vi "Write Tags.vi"(8 "error in (no error)":errorcluster, 10 "Array of Values":dbl[](array[numeric]), 11 "Communication Channel in":refnum<class "Communication Channel.lvclass">) -> (0 "error out":errorcluster, 3 "Communication Channel out":refnum<class "Communication Channel.lvclass">)   [LabVIEW 2014, in "Communication Channel.lvclass"]
uses:
  Communication Channel.lvclass
  Communication Channel.lvclass/Communication Channel.ctl
  <vilib>/Skyline/Tag/Wrapper/Wrapper_class/Write Tag (DBL).vi
  <vilib>/Skyline/Tag/Wrapper/Wrapper_class/NI Skyline Tag.lvclass
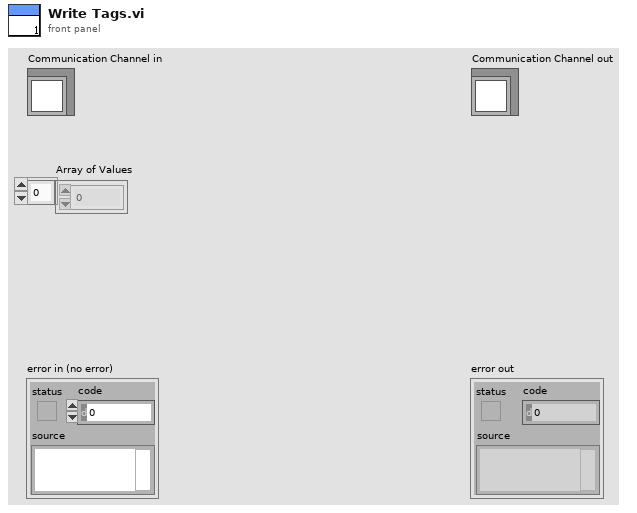
[diagram p1: front panel]
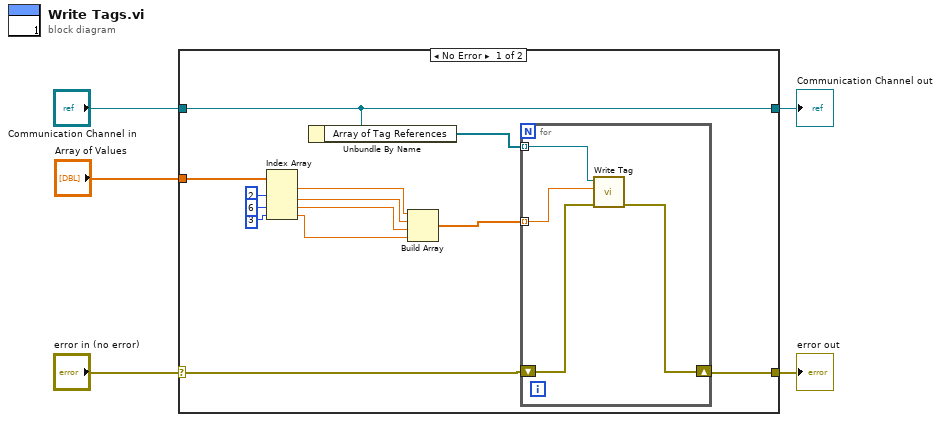
[diagram p0: block diagram]
diagram:
  n1 = case shown="No Error" "error in (no error)" {
    selector: "error in (no error)" -> [w16 w24]
    tunnel: [w15 w24] -> w4
    tunnel: [w17 w23] -> w2
    tunnel: "Communication Channel in" -> [w17 w23]
    tunnel: "Array of Values" -> [w18 _]
    frame No Error {
      n2 = Index Array(array=w18, index #2=2 ("index"), index #3=6 ("index"), index #4=3 ("index")) -> (element #1=w13:dbl, element #2=w11:dbl, element #3=w10:dbl, element #4=w7:dbl)  [unwired: 1 in]
      n3 = Unbundle By Name(w17) -> ("Array of Tag References"=w14:refnum<class "NI Skyline Tag.lvclass">[])
      n4 = Build Array(w13, w11, w10, w7) -> (w12:dbl[])
      n5 = for {
        shift-right: [w21] -> w15
        shift-left: w16 -> [w22]
        tunnel: w14 -> [w20] mode=indexing
        tunnel: w12 -> [w19] mode=indexing
        n6 = call-poly <vilib>:"Write Tag.vi"("error in (no error)"=w22, "value"=w19, "tag in"=w20) -> ("error out"=w21:errorcluster)  [unwired: 7 in, 1 out]
      }
    }
    frame Error {
    }
  }
  "error out" <- w4
  "Communication Channel out" <- w2
